vi "Exercise9.1-Basic Sine TX.vi"() -> ()   [LabVIEW 2013]
uses:
  <instrlib>/niUSRP/niUSRP Write Tx Data (CDB).vi
panel:
  out "error out":errorcluster
  out "coerced gain":dbl format="%#_6f"
  out "coerced carrier frequency":dbl=2400010000.007024 format="%#_6p"
  out "coerced IQ rate":dbl=200000.0 format="%#_6p"
  in  "Stop":bool
  in  "active antenna":string="TX1"
  in  "gain":dbl format="%#_6f"
  in  "carrier frequency":dbl=2400010000.0 format="%#_6p"
  in  "IQ rate":dbl=200000.0 format="%#_6p"
  in  "device names":refnum<k15>="192.168.10.2"
  in  "waveform size":i32=10000
  # "USRP Transmitter"
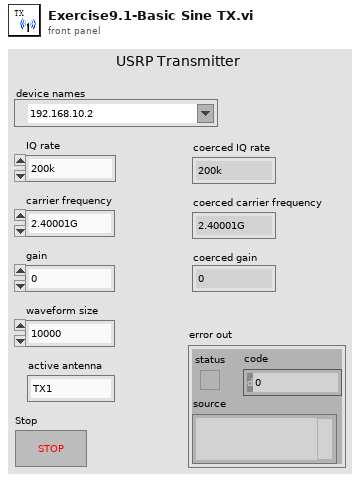
[diagram p1: front panel]
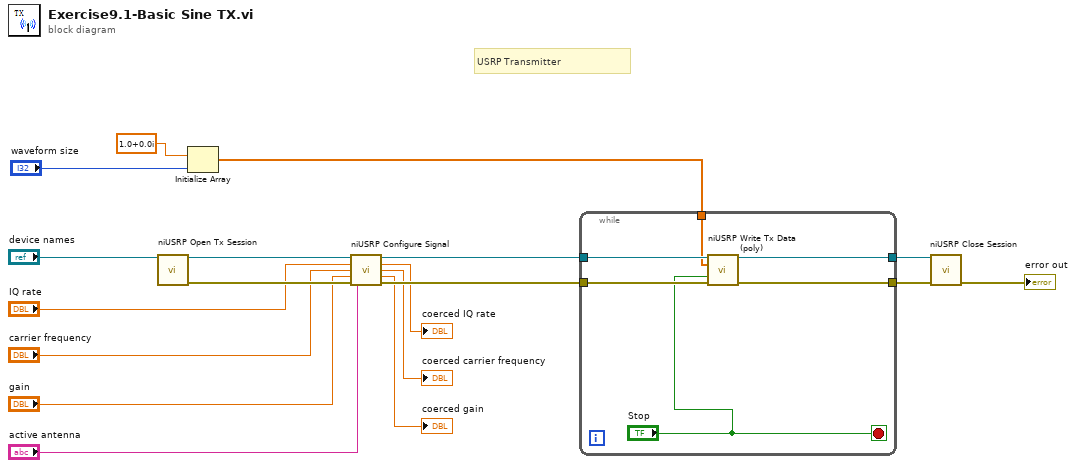
[diagram p0: block diagram]
diagram:
  # "USRP Transmitter"
  n1 = call <instrlib>:"niUSRP Open Tx Session.vi"("device names"="device names") -> ("session handle out"=w8:refnum<k15>, "error out"=w18:errorcluster)  [unwired: 13 in]
  n2 = Initialize Array "Initialize Array"(cdb 1.0+0.0i ("元素"), "waveform size") -> (w6:cdb[])
  n3 = call <instrlib>:"niUSRP Configure Signal.vi"("session handle"=w8, "IQ rate"="IQ rate", "carrier frequency"="carrier frequency", "gain"="gain", "error in (no error)"=w18, "active antenna"="active antenna") -> ("session handle out"=w7:refnum<k15>, "coerced IQ rate"=→"coerced IQ rate":dbl, "coerced carrier frequency"=→"coerced carrier frequency":dbl, "coerced gain"=→"coerced gain":dbl, "error out"=w17:errorcluster)  [unwired: 5 in]
  n4 = while {
    tunnel: w17 -> [w24]
    tunnel: [w23] -> w16
    tunnel: w7 -> [w22]
    tunnel: w6 -> [w20]
    tunnel: [w19] -> w5
    stop <- "Stop" stop-if-true
    n5 = call-poly <instrlib>:"niUSRP Write Tx Data (poly).vi"("session handle"=w22, "data"=w20, "end of data?"="Stop", "error in (no error)"=w24) -> ("session handle out"=w19:refnum<k15>, "error out"=w23:errorcluster)  [unwired: 10 in]
  }
  n6 = call <instrlib>:"niUSRP Close Session.vi"("session handle"=w5, "error in (no error)"=w16) -> ("error out"=→"error out":errorcluster)  [unwired: 13 in]
